vi "slide.vi"() -> ()   [LabVIEW 2018]
panel:
  out "Slide":u8(slide) scale=0.0..100.0
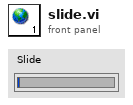
[diagram p1: front panel]
diagram:
